vi "send handshake response.vi"(9 "supported protocols":string[](array[string]), 10 "return sec key":string, 11 "TCP Network Connection in":refnum<k5>) -> (0 "error out":errorcluster)   [LabVIEW 2016, in "websocket standalone server.lvclass"]
uses:
  websocket standalone server.lvclass
  HTTP headers/http header data.ctl
  HTTP headers/http headers.lvlib
  HTTP server/http response packet type.ctl
  HTTP server/Basic HTTPS server.lvclass
  HTTP server/http response.ctl
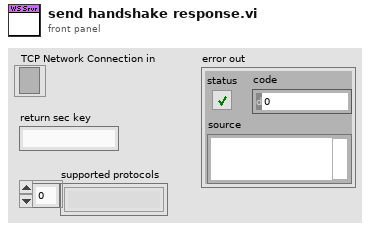
[diagram p1: front panel]
types:
  T1 = typedef "http headers.lvlib/http header data.ctl" = cluster{"lookup":variant}
  T2 = typedef "Basic HTTPS server.lvclass/http response packet type.ctl" = enum16{"full response", "header only", "data only", "last data", "raw output"}
  T3 = typedef "Basic HTTPS server.lvclass/http response.ctl" = cluster{"reason code":u16, "status string":string, "headers":T1, "cookies":string[], "data":string}
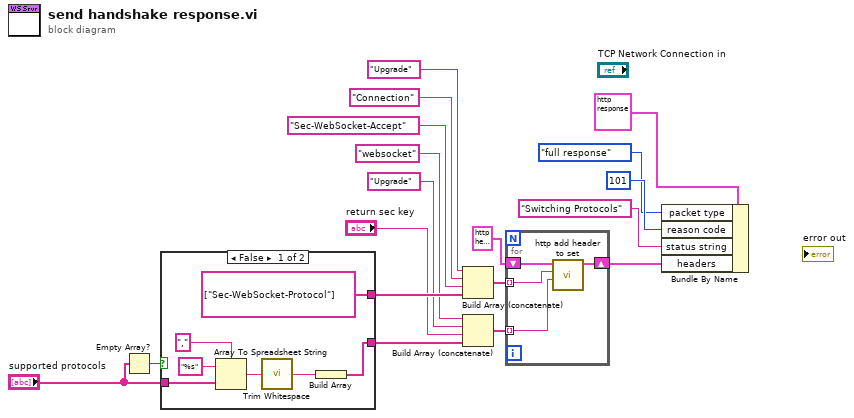
[diagram p0: block diagram]
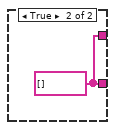
[diagram p2: hidden frame]
diagram:
  n1 = Empty Array?(array="supported protocols") -> (empty?=w16:bool)
  n2 = case shown="False" w16 {
    tunnel: [string[] ["Sec-WebSocket-Protocol"] ("appended array") w27] -> w17
    tunnel: [w24 w27] -> w18
    tunnel: "supported protocols" -> [w22 _]
    frame False {
      n3 = Array To Spreadsheet String(delimiter (Tab)=",", array=w22, 3:"%s" ("format string")) -> (spreadsheet string=w23:string)
      n4 = call <vilib>:"Trim Whitespace.vi"("string"=w23) -> ("trimmed string"=w25:string)  [unwired: 1 in]
      n5 = Build Array(w25) -> (w24:string[])
    }
    frame True {
      w27 = string[] [] ("appended array")
    }
  }
  n6 = Build Array (concatenate)("Upgrade" ("status string"), "Connection" ("status string"), "Sec-WebSocket-Accept" ("status string"), w17) -> (w3:string[])
  n7 = Build Array (concatenate)("websocket" ("status string"), "Upgrade" ("status string"), "return sec key", w18) -> (w2:string[])
  n8 = for {
    shift-right: [w31] -> w1
    shift-left: T1 {"lookup"=variant} ("headers out") -> [w30]
    tunnel: w3 -> [w29] mode=indexing
    tunnel: w2 -> [w28] mode=indexing
    n9 = call "http add header to set.vi"("header field data"=w28, "header field name"=w29, "headers in"=w30) -> ("headers out"=w31:T1)  [unwired: 8 in]
  }
  n10 = Bundle By Name(cluster=T3 {"reason code"=101, "status string"="", "headers"={"lookup"=variant}, "cookies"=[], "data"=""} ("application request"), "packet type"=http_response_packet_type."full response", "reason code"=u16 101, "status string"="Switching Protocols", "headers"=w1) -> ()  [unwired: 1 out]
